vi "Get Transform.vi"(8 "error in (no error)":errorcluster, 11 "Drawer .Net in":refnum<class "Drawer .Net.lvclass">) -> (0 "error out":errorcluster, 2 "Real Matrix 2x3":T1, 3 "Drawer .Net out":refnum<class "Drawer .Net.lvclass">)   [LabVIEW 2023, in "Glyph .NET Drawer.lvlib" / "Drawer .Net.lvclass"]
uses:
  Drawer .Net.lvclass
  <vilib>/Analysis/Matrix/Datatypes/RealMatrix.ctl
  Drawer .Net.lvclass/Drawer .Net.ctl
  System.Drawing
  <vilib>/Analysis/Matrix/NI_Matrix.lvlib
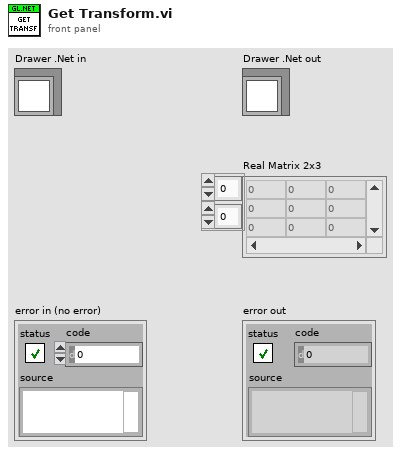
[diagram p1: front panel]
types:
  T1 = typedef "NI_Matrix.lvlib/RealMatrix.ctl" = dbl[][]
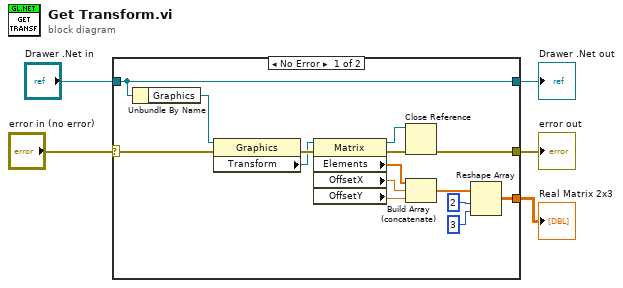
[diagram p0: block diagram]
diagram:
  n1 = case shown="No Error" "error in (no error)" {
    selector: "error in (no error)" -> [w18 w22]
    tunnel: [w14 w22] -> w4
    tunnel: [w20 w21] -> w2
    tunnel: "Drawer .Net in" -> [w20 w21]
    tunnel: [w6 _] -> w1
    frame No Error {
      n2 = Unbundle By Name(w20) -> ("Graphics"=w19:refnum<k24>)
      n3 = property class="Graphics"(reference=w19, error in=w18) -> (error out=w17:errorcluster, "Transform"=w15:refnum<k24>)  [unwired: 1 out]
      n4 = property class="Matrix"(reference=w15, error in=w17) -> (reference out=w13:refnum<k24>, error out=w16:errorcluster, "Elements"=w12:sgl[], "OffsetX"=w11:sgl, "OffsetY"=w10:sgl)
      n5 = Close Reference(reference=w13, error in (no error)=w16) -> (error out=w14:errorcluster)
      n6 = Build Array (concatenate)(w12, w11, w10) -> (w9:sgl[])
      n7 = Reshape Array(w9, 2 ("dimension size"), 3 ("dimension size")) -> (w6:sgl[][])
    }
    frame Error {
    }
  }
  "error out" <- w4
  "Drawer .Net out" <- w2
  "Real Matrix 2x3" <- w1
